vi "lia_fpga_chebyshev.vi"() -> ()   [LabVIEW 2009]
uses:
  <vilib>/eio/EIONode/EIONode.xnode
  <vilib>/rvi/eio/nirviEIOImplementation/nirviEIOImplementation.xnode
  <vilib>/rvi/eio/common/nirviEmuTemplateMethod_noerrors.vi
  <vilib>/rvi/eio/common/nirviEmuClasses.ctl
panel:
  in  "a1":i32[](array[numeric])=[0, 0, 0, 0, 0, 0]
  in  "b1":i32[](array[numeric])=[0, 0, 0, 0, 0, 0]
  out "XY_fpga":i32[](array[numeric])
  in  "a0":i32[](array[numeric])=[0, 0, 0, 0, 0, 0]
  in  "Signal Amplitude 3":u16
  in  "Phase Shift 3":u32
  in  "Accumulator Increment 3":u32
  in  "Signal Amplitude 2":u16
  in  "Phase Shift 2":u32
  in  "Accumulator Increment 2":u32
  in  "stop":bool
  out "Actual Gen Rate (ticks)":u32
  in  "Update Rate (ticks)":u32
  in  "Signal Amplitude 1":u16
  in  "Phase Shift 1":u32
  in  "Accumulator Increment 1":u32
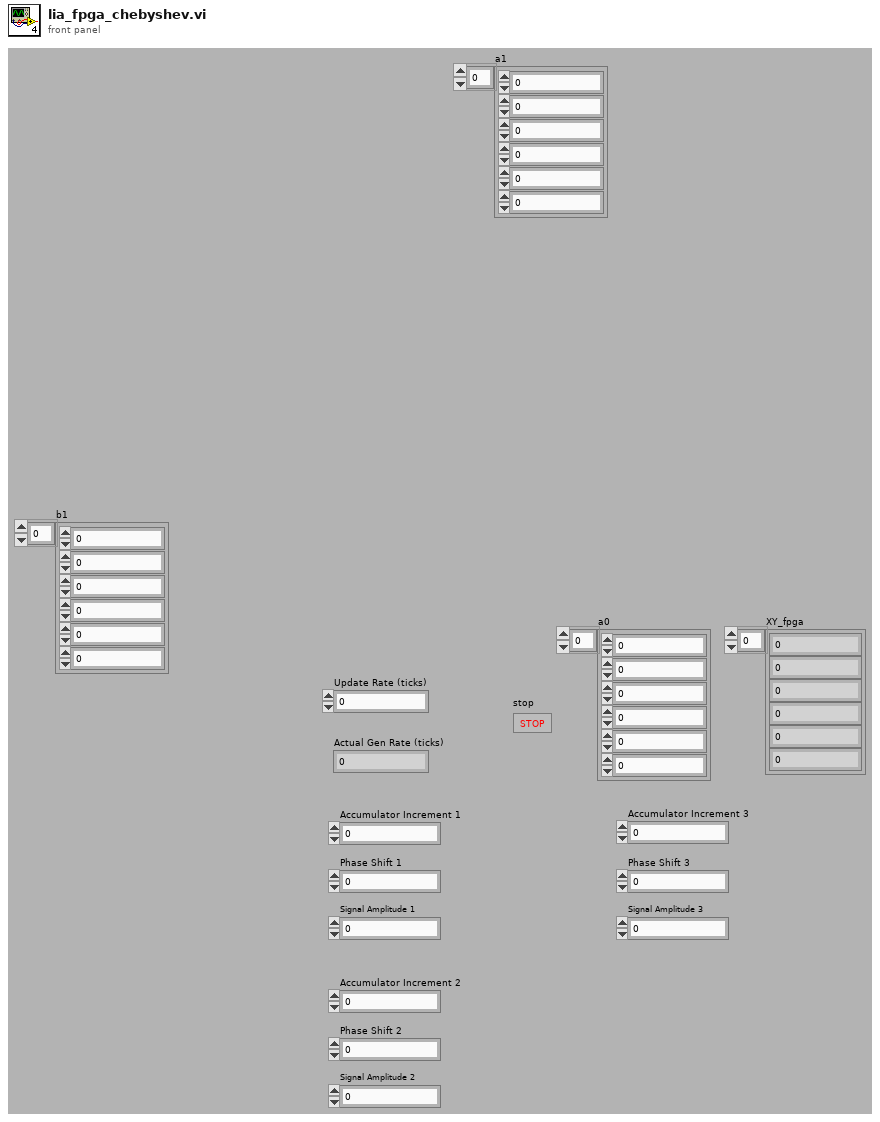
[diagram p1: front panel]
types:
  T1 = typedef "nirviEmuClasses.ctl" = enum16{"IO Read", "IO Write", "Method", "Property Read", "Property Write"}
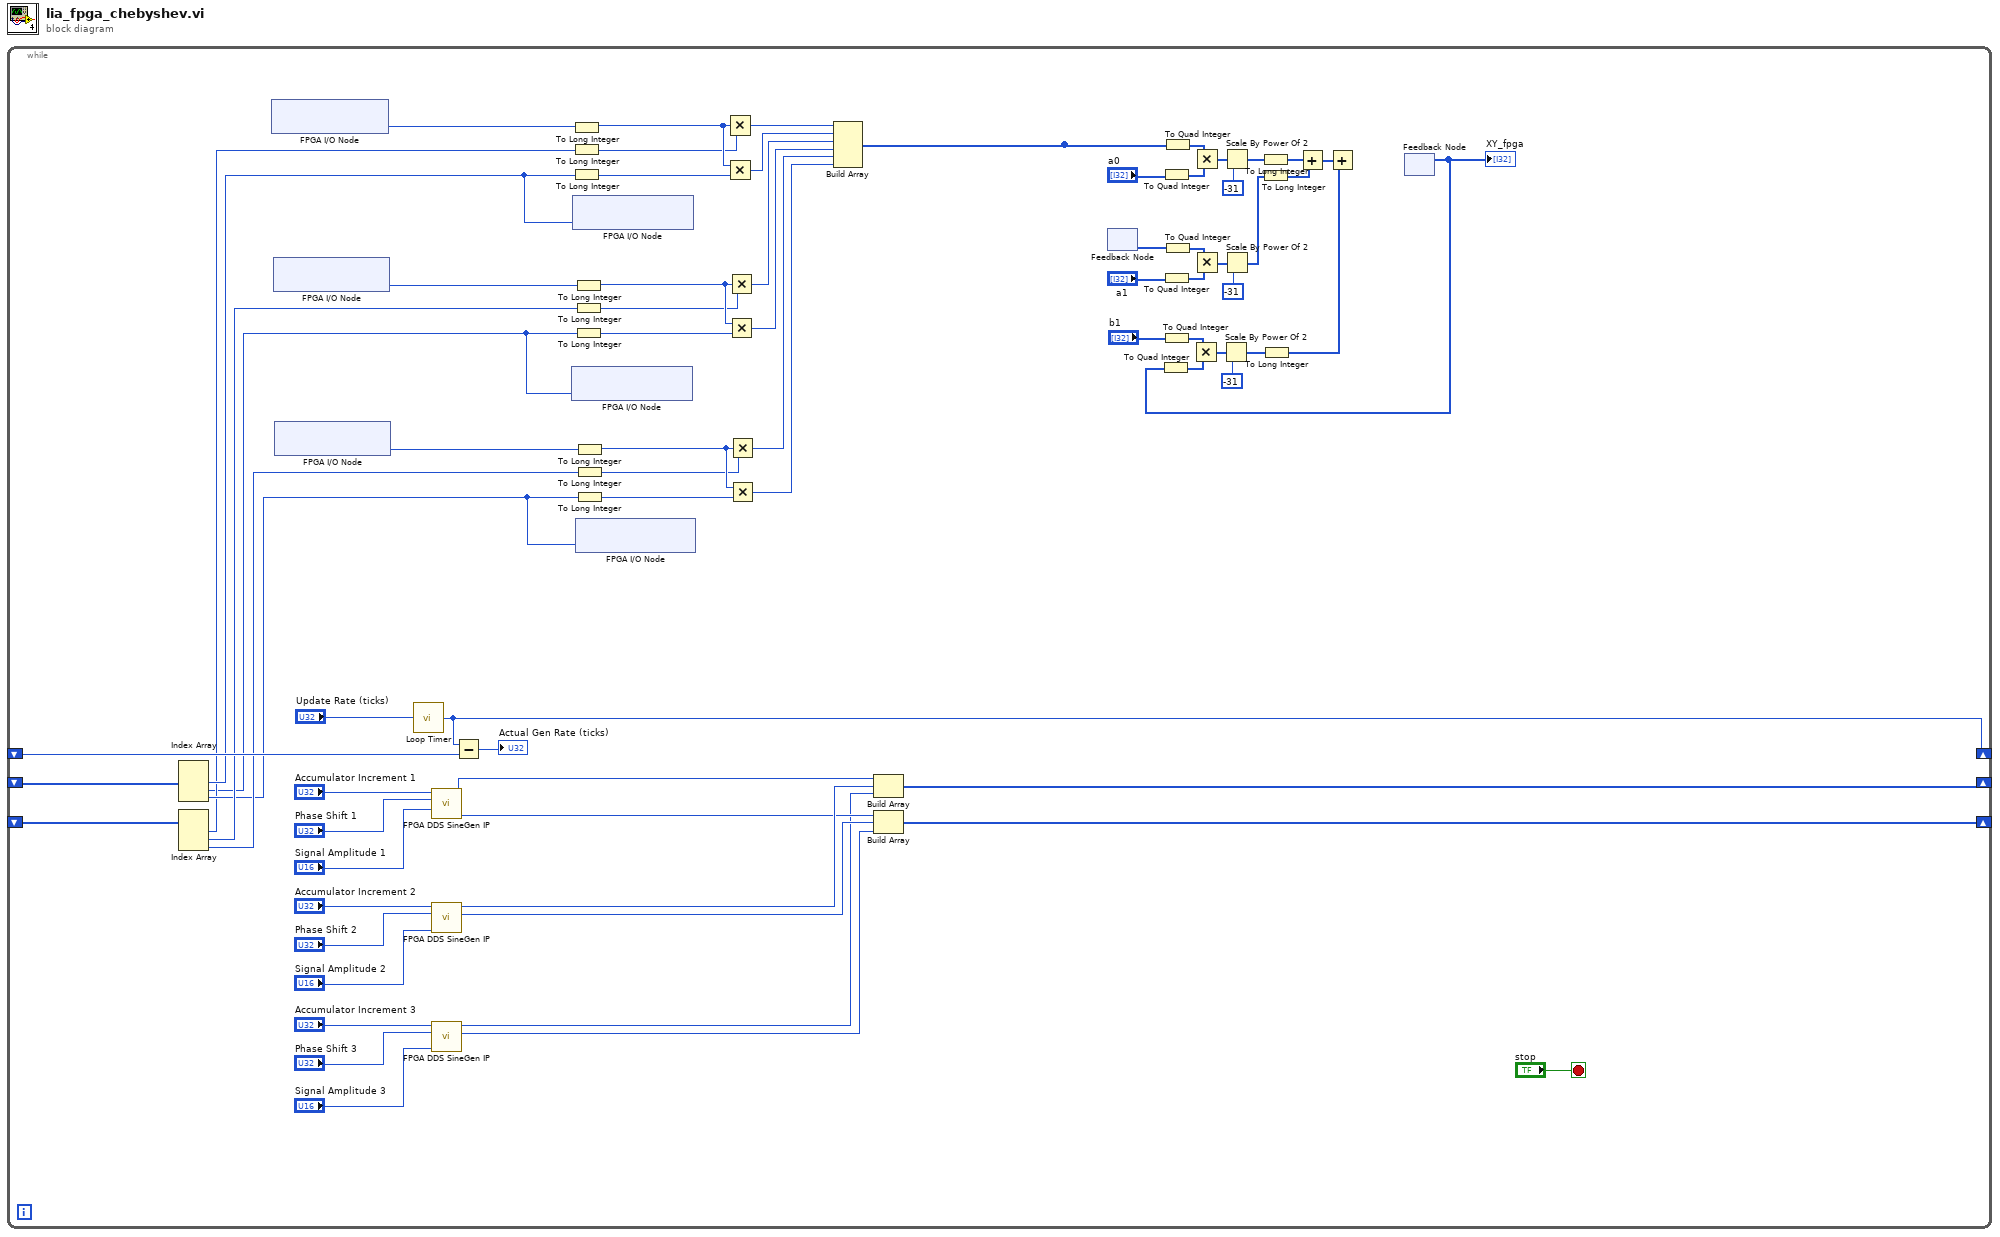
[diagram p0: block diagram]
diagram:
  n1 = while {
    shift-right: [w55] -> _
    shift-left: _ -> [w53]
    shift-right: [w71] -> _
    shift-left: _ -> [w69]
    shift-right: [w54] -> _
    shift-left: _ -> [w51]
    stop <- "stop" stop-if-true
    n2 = Index Array(array=w53) -> (element #1=w52:i16, element #2=w20:i16, element #3=w35:i16)  [unwired: 3 in]
    n3 = Index Array(array=w51) -> (element #1=w21:i16, element #2=w46:i16, element #3=w36:i16)  [unwired: 3 in]
    n4 = xnode "FPGA I/O Node"() -> ("Connector0/AI0"=w66:i16)  [unwired: 1 in, 1 out]
    n5 = xnode "FPGA I/O Node"() -> ("Connector0/AI1"=w50:i16)  [unwired: 1 in, 1 out]
    n6 = xnode "FPGA I/O Node"() -> ("Connector0/AI2"=w40:i16)  [unwired: 1 in, 1 out]
    n7 = call "Loop Timer"("Count(Ticks)"="Update Rate (ticks)") -> ("Tick Count(Ticks)"=w71:u32)
    n8 = call "FPGA DDS SineGen IP.vi"("Signal Amplitude (x 2^15)"="Signal Amplitude 1", "Phase Shift"="Phase Shift 1", "Accumulator Increment"="Accumulator Increment 1") -> ("Cos output"=w57:i16, "Sin output"=w59:i16)  [unwired: 6 in, 1 out]
    n9 = call "FPGA DDS SineGen IP.vi"("Signal Amplitude (x 2^15)"="Signal Amplitude 2", "Phase Shift"="Phase Shift 2", "Accumulator Increment"="Accumulator Increment 2") -> ("Cos output"=w56:i16, "Sin output"=w58:i16)  [unwired: 6 in, 1 out]
    n10 = call "FPGA DDS SineGen IP.vi"("Signal Amplitude (x 2^15)"="Signal Amplitude 3", "Phase Shift"="Phase Shift 3", "Accumulator Increment"="Accumulator Increment 3") -> ("Cos output"=w41:i16, "Sin output"=w42:i16)  [unwired: 6 in, 1 out]
    n11 = Subtract(x=w71, y=w69) -> (x-y=→"Actual Gen Rate (ticks)":u32)
    n12 = To Long Integer(number=w66) -> (32bit integer=w65:i32)
    n13 = To Long Integer(number=w21) -> (32bit integer=w64:i32)
    n14 = To Long Integer(number=w52) -> (32bit integer=w63:i32)
    n15 = xnode "FPGA I/O Node"("Connector0/AO1"=w20) -> ()  [unwired: 1 in, 1 out]
    n16 = xnode "FPGA I/O Node"("Connector0/AO0"=w52) -> ()  [unwired: 1 in, 1 out]
    n17 = To Long Integer(number=w50) -> (32bit integer=w49:i32)
    n18 = To Long Integer(number=w46) -> (32bit integer=w48:i32)
    n19 = To Long Integer(number=w20) -> (32bit integer=w47:i32)
    n20 = To Long Integer(number=w40) -> (32bit integer=w39:i32)
    n21 = To Long Integer(number=w36) -> (32bit integer=w38:i32)
    n22 = To Long Integer(number=w35) -> (32bit integer=w37:i32)
    n23 = xnode "FPGA I/O Node"("Connector0/AO2"=w35) -> ()  [unwired: 1 in, 1 out]
    n24 = Multiply(x=w65, y=w64) -> (x*y=w27:i32)
    n25 = Multiply(x=w65, y=w63) -> (x*y=w26:i32)
    n26 = Multiply(x=w49, y=w48) -> (x*y=w25:i32)
    n27 = Multiply(x=w49, y=w47) -> (x*y=w24:i32)
    n28 = Multiply(x=w39, y=w38) -> (x*y=w23:i32)
    n29 = Multiply(x=w39, y=w37) -> (x*y=w22:i32)
    n30 = Build Array(w27, w26, w25, w24, w23, w22) -> (w17:i32[])
    n31 = Build Array(w59, w58, w42) -> (w55:i16[])
    n32 = Build Array(w57, w56, w41) -> (w54:i16[])
    n33 = feedback #1() -> (w11:i32[])  [unwired: 1 in]
    n34 = To Quad Integer(1:"a0") -> (0:w31:i64[])
    n35 = To Quad Integer(1:"a1") -> (0:w13:i64[])
    n36 = To Quad Integer(1:"b1") -> (0:w29:i64[])
    n37 = To Quad Integer(1:w17) -> (0:w32:i64[])
    n38 = To Quad Integer(1:w11) -> (0:w14:i64[])
    n39 = Multiply(x=w32, y=w31) -> (x*y=w34:i64[])
    n40 = Multiply(x=w14, y=w13) -> (x*y=w16:i64[])
    n41 = Scale By Power Of 2(n=i16 -31, x=w34) -> (x*2^n=w4:i64[])
    n42 = Scale By Power Of 2(n=i16 -31, x=w16) -> (x*2^n=w5:i64[])
    n43 = To Long Integer(number=w4) -> (32bit integer=w3:i32[])
    n44 = To Long Integer(number=w5) -> (32bit integer=w2:i32[])
    n45 = Add(x=w3, y=w2) -> (x+y=w10:i32[])
    n46 = feedback #2() -> (w1:i32[])  [unwired: 1 in]
    "XY_fpga" <- w1
    n47 = To Quad Integer(1:w1) -> (0:w28:i64[])
    n48 = Multiply(x=w29, y=w28) -> (x*y=w30:i64[])
    n49 = Scale By Power Of 2(n=i16 -31, x=w30) -> (x*2^n=w7:i64[])
    n50 = To Long Integer(number=w7) -> (32bit integer=w6:i32[])
    n51 = Add(x=w10, y=w6) -> (x+y=w9:i32[])
  }
